vi "Open VI and BD.vi"(7 "App":refnum<vi>, 8 "error in (no error)":errorcluster, 11 "VI Path":path) -> (0 "error out":errorcluster, 2 "BD":refnum<vi>, 3 "VI":refnum<vi>)   [LabVIEW 2020, in "LV-Protoc.lvlib"]
uses:
  LV-Protoc.lvlib
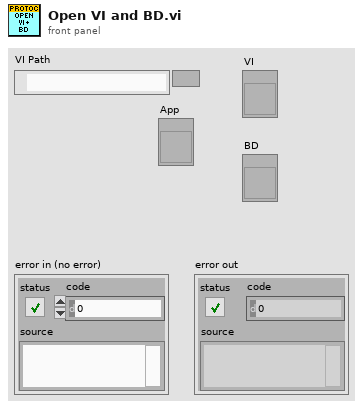
[diagram p1: front panel]
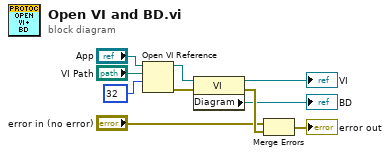
[diagram p0: block diagram]
diagram:
  n1 = Open VI Reference(application reference (local)="App", vi path="VI Path", options=32) -> (vi reference=w8:refnum<vi>, error out=w9:errorcluster)  [unwired: 3 in]
  n2 = property class="VI"(reference=w8, error in=w9) -> (reference out=→"VI":refnum<vi>, error out=w10:errorcluster, "Diagram"=→"BD":refnum<vi>)
  n3 = Merge Errors("error in (no error)", w10) -> (→"error out":errorcluster)
